vi "Layer Scan V5.vi"() -> ()   [LabVIEW 2024]
uses:
  <vilib>/DAQmx/write.llb/DAQmx Write (Analog 1D DBL NChan 1Samp).vi
  <vilib>/DAQmx/create/channels.llb/DAQmx Create Channel (AO-Voltage-Basic).vi
  <vilib>/DAQmx/miscellaneous.llb/DAQmx Fill In Error Info.vi
  <instrlib>/niScope/Utility/niScope Get Channel Name From String.vi
  <instrlib>/niScope/Configure/Trigger/niScope Configure Trigger Immediate.vi
  <instrlib>/niScope/Configure/Trigger/niScope Configure Trigger Edge.vi
  <instrlib>/niScope/Configure/Trigger/niScope Configure Trigger Digital.vi
  <instrlib>/niScope/Configure/Trigger/niScope Configure Trigger Window.vi
  <instrlib>/niScope/Configure/Trigger/niScope Configure Trigger Hysteresis.vi
  <instrlib>/niScope/Acquire/Fetch/niScope Multi Fetch.vi
panel:
  in  "Resource Name":refnum<k15>="Dev1" caption="Resource Name(s)"
  in  "Simulate?":bool
  in  "Channel Name":string="0" caption="Channel(s)"
  in  "Enforce Realtime":bool=TRUE
  in  "Vertical Range":dbl=5.0 caption="Vertical Range (V)" format="%.2f"
  in  "Min Sample Rate":dbl=10000000.0 caption="Min. Sample Rate" step=1000000.0 format="%#.2p"
  in  "Min Record Length":i32=1000 caption="Min. Record Length"
  out "Waveform(s)":dbl[][](graph)
  out "Actual Record Length":i32=1000
  out "Actual Sample Rate":dbl=10000000.0 format="%#.2p"
  in  "Timeout (s)":dbl=5.0 caption="Timeout(s)" format="%.2f"
  in  "Vertical Offset":dbl caption="Vertical Offset (V)" format="%.2p"
  in  "Probe Attenuation":dbl=1.0 format="%.1f"
  in  "Input Impedance":u32(ring) items=["1 mega ohm"=0, "50 ohms"=2]
  in  "Maximum Input Frequency":dbl caption="Max. Input Frequency (Hz)" format="%.2f"
  in  "Trigger Delay":dbl caption="Trigger Delay (s)" format="%#.4p"
  in  "Reference Position":dbl=50.0 caption="Ref Position" format="%.1f"
  in  "Stop":bool
  in  "Vertical Coupling":i32(ring)=1 items=["AC", "DC", "Ground"]
  in  "Trigger Modifier":i32(ring)=2 items=["None"=1, "Auto Trigger"=2]
  out "Auto Triggered":bool
  in  "Trigger Type":T1(tab)
  in  "Trigger Source":string(combo)="0"
  in  "Trigger Level":dbl format="%.2f"
  in  "Trigger Slope":i32(ring) items=["Positive", "Negative"]
  in  "Coupling":u16(ring)=1 caption="Trigger Coupling" items=["AC"=0, "DC"=1, "HF Reject"=3, "LF Reject"=4, "AC Plus HF Reject"=1001]
  in  "Trigger Slope 2":i32(ring) caption="Trigger Slope" items=["Positive", "Negative"]
  in  "Trigger Source 2":string(combo)="VAL_PFI_1" caption="Trigger Source"
  in  "Coupling 2":u16(ring)=1 caption="Trigger Coupling" items=["AC"=0, "DC"=1, "HF Reject"=3, "LF Reject"=4, "AC Plus HF Reject"=1001]
  in  "High Level":dbl=0.1 caption="Window High Level" format="%.2f"
  in  "Low Level":dbl=-0.1 caption="Window Low Level" format="%.2f"
  in  "Window Mode":i32(ring) items=["Entering", "Leaving"]
  in  "Trigger Source 3":string(combo)="0" caption="Trigger Source"
  in  "Hysteresis":dbl=0.05 format="%.2f"
  in  "Trigger Source 4":string(combo)="0" caption="Trigger Source"
  in  "Trigger Level 2":dbl caption="Trigger Level" format="%.2f"
  in  "Coupling 3":u16(ring)=1 caption="Trigger Coupling" items=["AC"=0, "DC"=1, "HF Reject"=3, "LF Reject"=4, "AC Plus HF Reject"=1001]
  in  "Trigger Slope 3":i32(ring) caption="Trigger Slope" items=["Positive", "Negative"]
  out "decimated array 2":dbl[](array[numeric])
  out "decimated array":dbl[](array[numeric])
  out "Y coord filename":i32
  out "x coord file name":i32
  out "Filename Out":path
  in  "Data File Name":path
  in  "Data folder Path":path
  in  "X offset":dbl
  in  "Y offset":dbl
  in  "distance":dbl
  in  "Y Count":dbl
  in  "X Count":dbl
  # "Note: When configured for Immediate reference trigger, this example does not configure any additional trigger settings - the acquisition is triggered as soon as possible after being initiated by driver software."
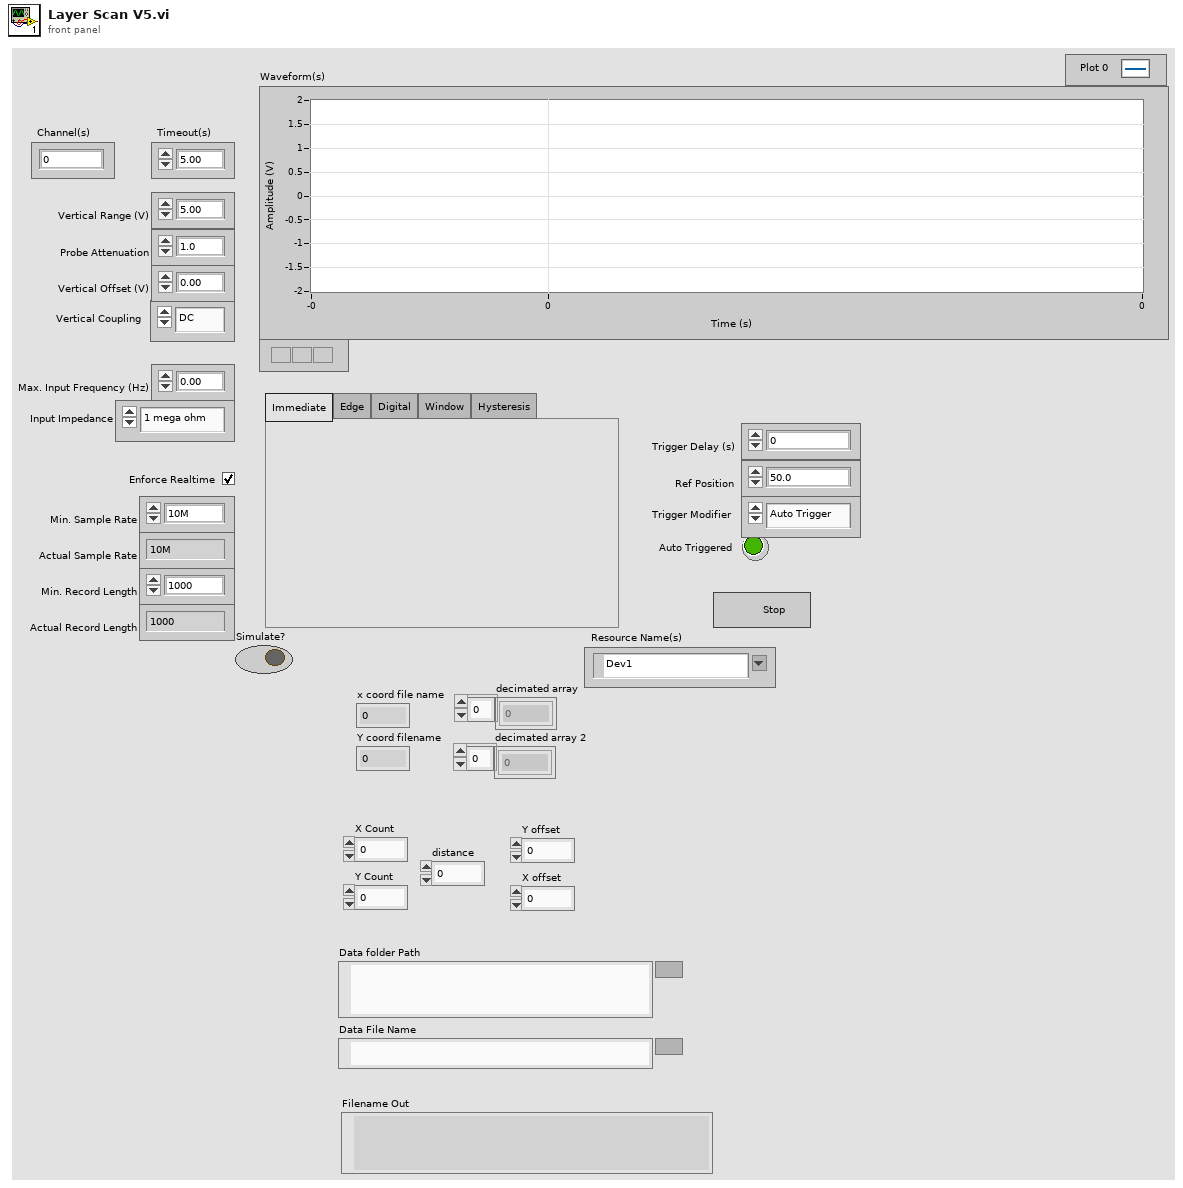
[diagram p1: front panel]
types:
  T1 = enum32{"Immediate", "Edge", "Digital", "Window", "Hysteresis"}
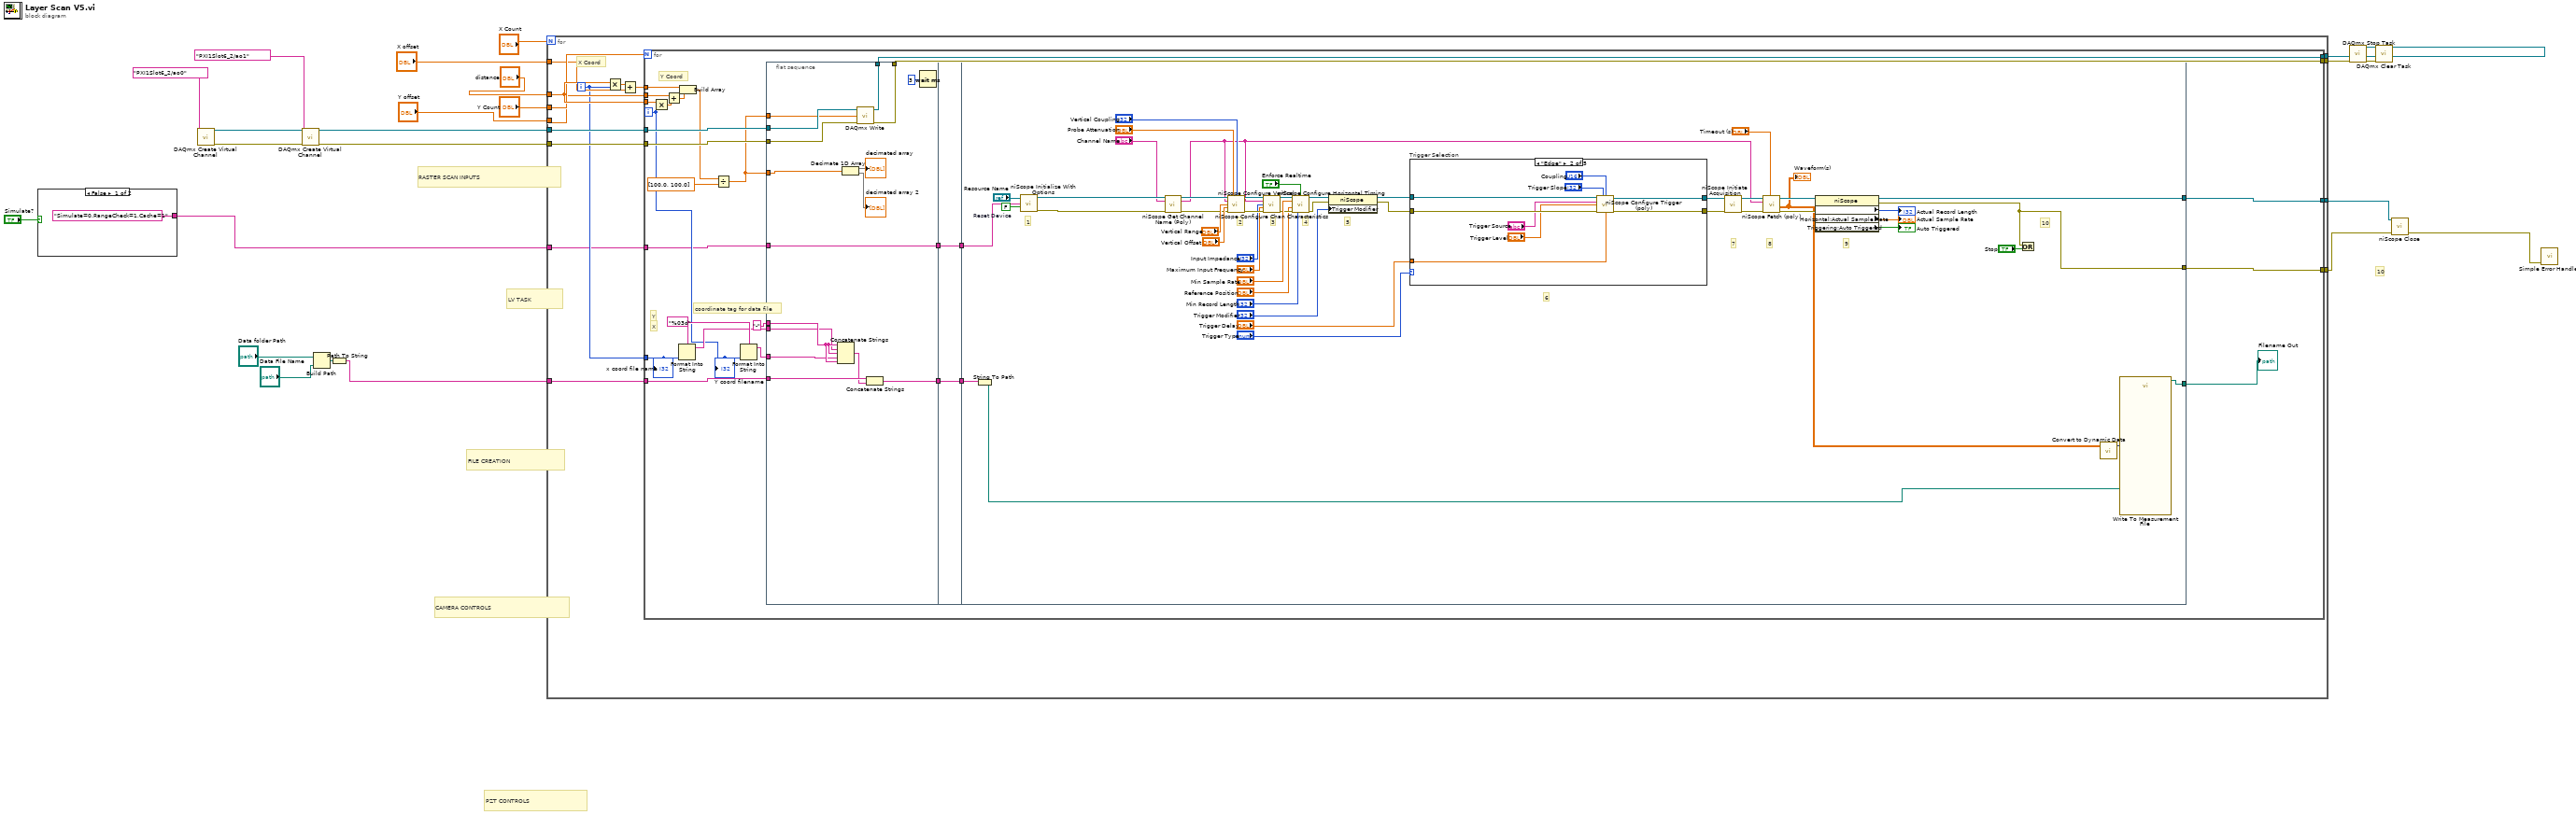
[diagram p0: block diagram]
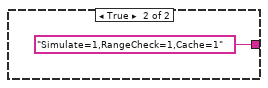
[diagram p2: hidden frame]
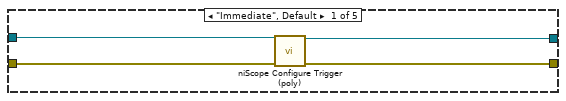
[diagram p3: hidden frame]
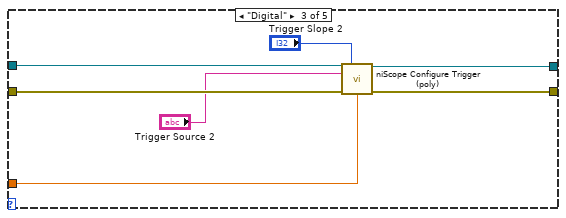
[diagram p4: hidden frame]
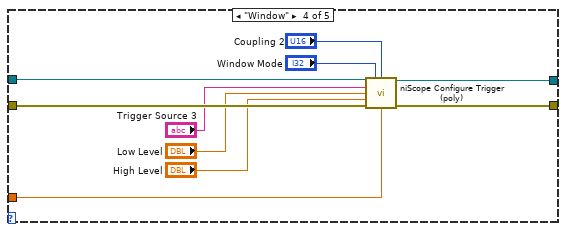
[diagram p5: hidden frame]
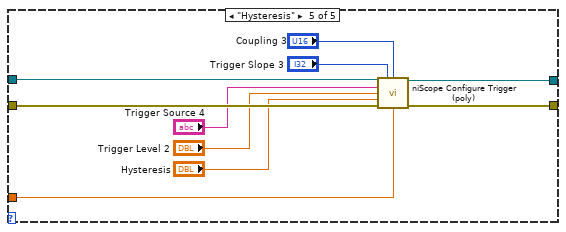
[diagram p6: hidden frame]
diagram:
  # "10"
  # "FILE CREATION"
  # "PZT CONTROLS"
  # "CAMERA CONTROLS"
  # "LV TASK"
  # "RASTER SCAN INPUTS"
  n1 = case shown="False" "Simulate?" {
    tunnel: ["Simulate=0,RangeCheck=1,Cache=1" ("option string") "Simulate=1,RangeCheck=1,Cache=1" ("option string")] -> w1
    frame False {
    }
    frame True {
    }
  }
  n2 = call-poly <vilib>:"DAQmx Create Virtual Channel.vi"("physical channels"=tag "PXI1Slot6_2/ao0") -> ("task out"=w17:refnum<k21>, "error out"=w16:errorcluster)  [unwired: 13 in]
  n3 = call-poly <vilib>:"DAQmx Create Virtual Channel.vi"("task in"=w17, "physical channels"=tag "PXI1Slot6_2/ao1", "error in"=w16) -> ("task out"=w15:refnum<k21>, "error out"=w14:errorcluster)  [unwired: 11 in]
  n4 = Build Path(base path="Data folder Path", name or relative path="Data File Name") -> (appended path=w7:path)
  n5 = Path To String(path=w7) -> (string=w6:string)
  n6 = for {
    N: "X Count" -> [_]
    tunnel: "distance" -> [w41]
    tunnel: "Y Count" -> [w40]
    tunnel: "Y offset" -> [w39]
    tunnel: "X offset" -> [w37]
    tunnel: w15 -> [w35]
    tunnel: w14 -> [w34]
    tunnel: [w33] -> w13
    tunnel: [w32] -> w12
    tunnel: [w31] -> w4
    tunnel: w6 -> [w30]
    tunnel: w1 -> [w28]
    tunnel: [w27] -> w5
    i -> [w29]
    # "X Coord"
    n7 = Multiply(x=w41, y=w29) -> (x*y=w38:dbl)
    n8 = Add(x=w38, y=w37) -> (x+y=w36:dbl)
    n9 = for {
      N: w40 -> [_]
      tunnel: w41 -> [w68]
      tunnel: w39 -> [w66]
      tunnel: w36 -> [w65]
      tunnel: w35 -> [w63]
      tunnel: w34 -> [w62]
      tunnel: [w60] -> w33
      tunnel: [w59] -> w32
      tunnel: [w47] -> w31
      tunnel: w30 -> [w54]
      tunnel: w29 -> [w50]
      tunnel: w28 -> [w43]
      tunnel: [w42] -> w27
      i -> [w49]
      w58 = "%03d" ("format string")
      # "coordinate tag for data file"
      # "X"
      # "Y"
      # "Y Coord"
      n10 = Multiply(x=w68, y=w49) -> (x*y=w67:dbl)
      n11 = Add(x=w66, y=w67) -> (x+y=w64:dbl)
      n12 = Format Into String(format string=w58, w50) -> (resulting string=w56:string)  [unwired: 2 in, 1 out]
      n13 = Build Array(w65, w64) -> (w61:dbl[])
      n14 = Divide(x=w61, y=dbl[] [100.0, 100.0]) -> (x/y=w48:dbl[])
      n15 = Format Into String(format string=w58, w49) -> (resulting string=w55:string)  [unwired: 2 in, 1 out]
      n16 = flat-sequence {
        tunnel: w63 -> [w83]
        tunnel: w62 -> [w82]
        tunnel: [w81] -> w60
        tunnel: [w80] -> w59
        tunnel: "-" ("string") -> [w79]
        tunnel: w56 -> [w78]
        tunnel: w55 -> [w77]
        tunnel: w54 -> [w76]
        tunnel: [w74] -> w53
        tunnel: w48 -> [w73]
        tunnel: w48 -> [w72]
        tunnel: [w69] -> w45
        tunnel: w43 -> [w69]
        tunnel: w53 -> [w86]
        tunnel: [w86] -> w52
        tunnel: w45 -> [w85]
        tunnel: [w85] -> w44
        tunnel: w52 -> [w126]
        tunnel: [w133] -> w47
        tunnel: [w134] -> w46
        tunnel: w44 -> [w128]
        tunnel: [w132] -> w42
        frame #0 {
          n17 = Concatenate Strings(w79, w78, w79, w77, w79) -> (w75:string)
          n18 = Decimate 1D Array(w72) -> (→"decimated array":dbl[], →"decimated array 2":dbl[])
          n19 = call-poly <vilib>:"DAQmx Write.vi"("task/channels in"=w83, "data"=w73, "error in"=w82) -> ("task out"=w81:refnum<k21>, "error out"=w80:errorcluster)  [unwired: 10 in, 1 out]
          n20 = Concatenate Strings(w76, w75) -> (w74:string)
          n21 = Wait (ms)(milliseconds to wait=u32 3) -> ()  [unwired: 1 out]
        }
        frame #1 {
        }
        frame #2 {
          w131 = FALSE  # Reset Device
          # "5"
          # "2"
          # "3"
          # "4"
          # "6"
          # "7"
          # "8"
          # "9"
          # "10"
          # "1"
          n22 = String To Path(string=w126) -> (path=w125:path)
          n23 = call <instrlib>:"niScope Initialize With Options.vi"("resource name"="Resource Name", "option string"=w128, "reset device"=w131) -> ("instrument handle"=w127:refnum<k15>, "error out"=w129:errorcluster)  [unwired: 11 in]
          n24 = call-poly <instrlib>:"niScope Get Channel Name (Poly).vi"("instrument handle"=w127, "index"="Channel Name", "error in"=w129) -> ("instrument handle out"=w92:refnum<k15>, "channel name"=w89:string, "error out"=w91:errorcluster)  [unwired: 10 in]
          n25 = call <instrlib>:"niScope Configure Vertical.vi"("instrument handle"=w92, "probe attenuation"="Probe Attenuation", "vertical coupling"="Vertical Coupling", "channels"=w89, "vertical range"="Vertical Range", "vertical offset"="Vertical Offset", "error in"=w91) -> ("instrument handle out"=w121:refnum<k15>, "error out"=w120:errorcluster)  [unwired: 7 in]
          n26 = call <instrlib>:"niScope Configure Chan Characteristics.vi"("instrument handle"=w121, "channels"=w89, "input impedance"="Input Impedance", "maximum input frequency"="Maximum Input Frequency", "error in"=w120) -> ("instrument handle out"=w118:refnum<k15>, "error out"=w119:errorcluster)  [unwired: 9 in]
          n27 = call <instrlib>:"niScope Configure Horizontal Timing.vi"("instrument handle"=w118, "enforce realtime"="Enforce Realtime", "min sample rate"="Min Sample Rate", "reference position"="Reference Position", "error in"=w119, "min record length"="Min Record Length") -> ("instrument handle out"=w104:refnum<k15>, "error out"=w103:errorcluster)  [unwired: 8 in]
          n28 = property on="Property Node" class="niScope"(reference=w104, error in=w103, "Trigger Modifier"="Trigger Modifier") -> (reference out=w101:refnum<k15>, error out=w102:errorcluster)
          n29 = case "Trigger Selection" shown="\"Edge\"" "Trigger Type" {
            tunnel: w102 -> [w138 w147 w154 w164 w174]
            tunnel: [w135 w143 w150 w160 w170] -> w107
            tunnel: w101 -> [w137 w146 w153 w163 w173]
            tunnel: [w136 w144 w151 w161 w172] -> w110
            tunnel: "Trigger Delay" -> [_ w145 w152 w162 w171]
            frame "Immediate", Default {
              n30 = call-poly <instrlib>:"niScope Configure Trigger (poly).vi"("instrument handle"=w137, "error in"=w138) -> ("instrument handle out"=w136:refnum<k15>, "error out"=w135:errorcluster)  [unwired: 12 in]
            }
            frame "Edge" {
              n31 = call-poly <instrlib>:"niScope Configure Trigger (poly).vi"("instrument handle"=w146, "trigger slope"="Trigger Slope", "trigger coupling"="Coupling", "trigger source"="Trigger Source", "trigger level"="Trigger Level", "error in"=w147, "trigger delay"=w145) -> ("instrument handle out"=w144:refnum<k15>, "error out"=w143:errorcluster)  [unwired: 7 in]
            }
            frame "Digital" {
              n32 = call-poly <instrlib>:"niScope Configure Trigger (poly).vi"("instrument handle"=w153, "trigger slope"="Trigger Slope 2", "trigger source"="Trigger Source 2", "error in"=w154, "trigger delay"=w152) -> ("instrument handle out"=w151:refnum<k15>, "error out"=w150:errorcluster)  [unwired: 9 in]
            }
            frame "Window" {
              n33 = call-poly <instrlib>:"niScope Configure Trigger (poly).vi"("instrument handle"=w163, "trigger window mode"="Window Mode", "trigger coupling"="Coupling 2", "trigger source"="Trigger Source 3", "low level"="Low Level", "high level"="High Level", "error in"=w164, "trigger delay"=w162) -> ("instrument handle out"=w161:refnum<k15>, "error out"=w160:errorcluster)  [unwired: 6 in]
            }
            frame "Hysteresis" {
              n34 = call-poly <instrlib>:"niScope Configure Trigger (poly).vi"("instrument handle"=w173, "trigger slope"="Trigger Slope 3", "trigger coupling"="Coupling 3", "trigger source"="Trigger Source 4", "trigger level"="Trigger Level 2", "hysteresis"="Hysteresis", "error in"=w174, "trigger delay"=w171) -> ("instrument handle out"=w172:refnum<k15>, "error out"=w170:errorcluster)  [unwired: 6 in]
            }
          }
          n35 = call <instrlib>:"niScope Initiate Acquisition.vi"("instrument handle"=w110, "error in"=w107) -> ("instrument handle out"=w109:refnum<k15>, "error out"=w108:errorcluster)  [unwired: 12 in]
          n36 = call-poly <instrlib>:"niScope Fetch (poly).vi"("timeout"="Timeout (s)", "error in"=w108, "channels"=w89, "instrument handle"=w109) -> ("error out"=w98:errorcluster, "wfm"=w88:dbl[][], "instrument handle out"=w99:refnum<k15>)  [unwired: 4 in, 1 out]
          "Waveform(s)" <- w88
          n37 = property class="niScope"(reference=w99, error in=w98) -> (reference out=w132:refnum<k15>, error out=w133:errorcluster, "Horizontal:Actual Record Length"=→"Actual Record Length":i32, "Horizontal:Actual Sample Rate"=→"Actual Sample Rate":dbl, "Triggering:Auto Triggered"=→"Auto Triggered":bool)
          n38 = Or(x=w133, y="Stop") -> ()  [unwired: 1 out]
          n39 = call "Convert to Dynamic Data"("2D Array"=w88) -> ("Dynamic Data Type"=w87:dynamicdata)  [unwired: 3 in]
          n40 = call "Write To Measurement File"("Signals"=w87, "Filename"=w125) -> ("Filename Out"=w134:path)  [unwired: 15 in, 2 out]
        }
      }
      "Filename Out" <- w46
      "x coord file name" <- w50
      "Y coord filename" <- w49
    }
  }
  n41 = call <vilib>:"DAQmx Stop Task.vi"("task/channels in"=w13, "error in"=w12) -> ("task out"=w11:refnum<k21>, "error out"=w10:errorcluster)  [unwired: 12 in]
  n42 = call <vilib>:"DAQmx Clear Task.vi"("task in"=w11, "error in"=w10) -> ()  [unwired: 13 in, 1 out]
  n43 = call <instrlib>:"niScope Close.vi"("instrument handle"=w5, "error in"=w4) -> ("error out"=w3:errorcluster)  [unwired: 13 in]
  n44 = call <vilib>:"Simple Error Handler.vi"("error in (no error)"=w3) -> ()  [unwired: 4 in, 5 out]
